vi "Test4.vi"() -> ()   [LabVIEW 2010]
uses:
  <vilib>/MDSplus/Library/MDSplus.lvlib
panel:
  out "Float out":sgl
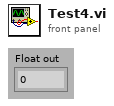
[diagram p1: front panel]
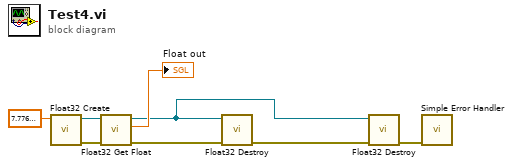
[diagram p0: block diagram]
diagram:
  n1 = call <vilib>:"Float32 Create.vi"("SGL in"=sgl 7.777 ("Value")) -> ("error out"=w6:errorcluster, "Float32 DVR out"=w7:refnum<data-value>)  [unwired: 9 in]
  n2 = call <vilib>:"Float32 Get Float.vi"("error in (no error)"=w6, "Float32 DVR in"=w7) -> ("error out"=w2:errorcluster, "SGL out"=→"Float out":sgl, "Float32 DVR out"=w3:refnum<data-value>)  [unwired: 6 in]
  n3 = call <vilib>:"Float32 Destroy.vi"("error in (no error)"=w2, "Scalar DVR in"=w3) -> ("error out"=w1:errorcluster)  [unwired: 8 in]
  n4 = call <vilib>:"Float32 Destroy.vi"("error in (no error)"=w1, "Scalar DVR in"=w3) -> ("error out"=w4:errorcluster)  [unwired: 8 in]
  n5 = call <vilib>:"Simple Error Handler.vi"("error in (no error)"=w4) -> ()  [unwired: 4 in, 5 out]
